vi "Cooling system dashboard.vi"() -> ()   [LabVIEW 2022 SP3]
uses:
  <vilib>/Instr/_visa.llb/VISA Configure Serial Port (Instr).vi
panel:
  out "array":dbl[](array[numeric])
  in  "stop":bool
  out "read buffer":string
  in  "baud rate (9600)":u32=9600
  in  "VISA resource name":refnum<visa-resource-name>
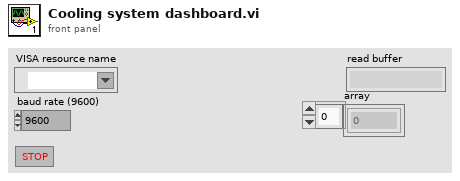
[diagram p1: front panel]
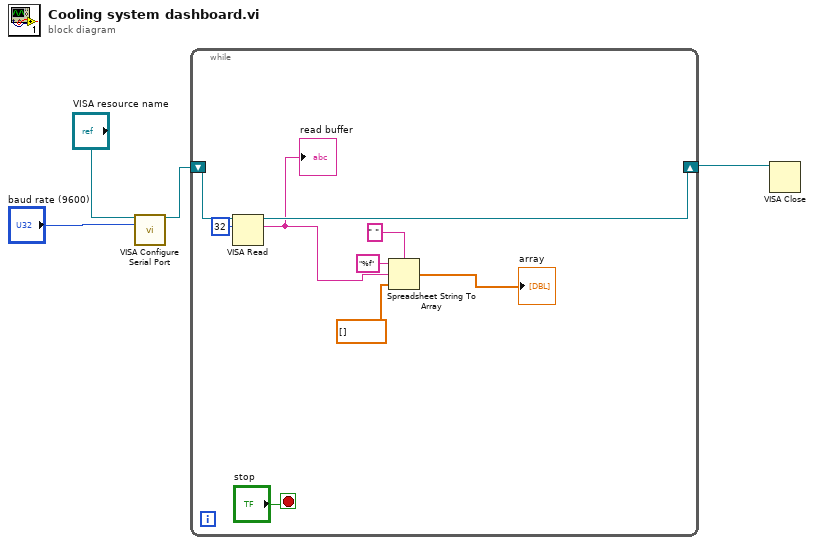
[diagram p0: block diagram]
diagram:
  n1 = call-poly "VISA Configure Serial Port"("VISA resource name"="VISA resource name", "baud rate (9600)"="baud rate (9600)") -> ("VISA resource name out"=w4:refnum<visa-resource-name>)  [unwired: 12 in, 1 out]
  n2 = while {
    shift-right: [w12] -> w1
    shift-left: w4 -> [w13]
    stop <- "stop" stop-if-true
    n3 = VISA Read(VISA resource name=w13, byte count=u32 32) -> (VISA resource name out=w12:refnum<visa-resource-name>, read buffer=w7:string)  [unwired: 1 in, 2 out]
    "read buffer" <- w7
    n4 = Spreadsheet String To Array(delimiter (Tab)=" ", format string="%f", spreadsheet string=w7, array type (2D Dbl)=dbl[] []) -> (array=→"array":dbl[])
  }
  n5 = VISA Close(VISA resource name=w1) -> ()  [unwired: 1 in, 1 out]
